vi "PlLoN_grabber.vi"(7 "Number of Images":u32=1 min=1 step=1, 8 "error in (no error)":errorcluster, 11 "Camera Handle":u32) -> (0 "error out":errorcluster, 1 "DATA":u16[][](array[numeric]), 2 "Number of Images":u32=1 min=1 step=1, 3 "Camera Handle":u32, 4 "x/y":dbl)   [LabVIEW 2015]
panel:
  out "Waveform Graph":u16[][](graph)
  out "PyLoN Ready":bool
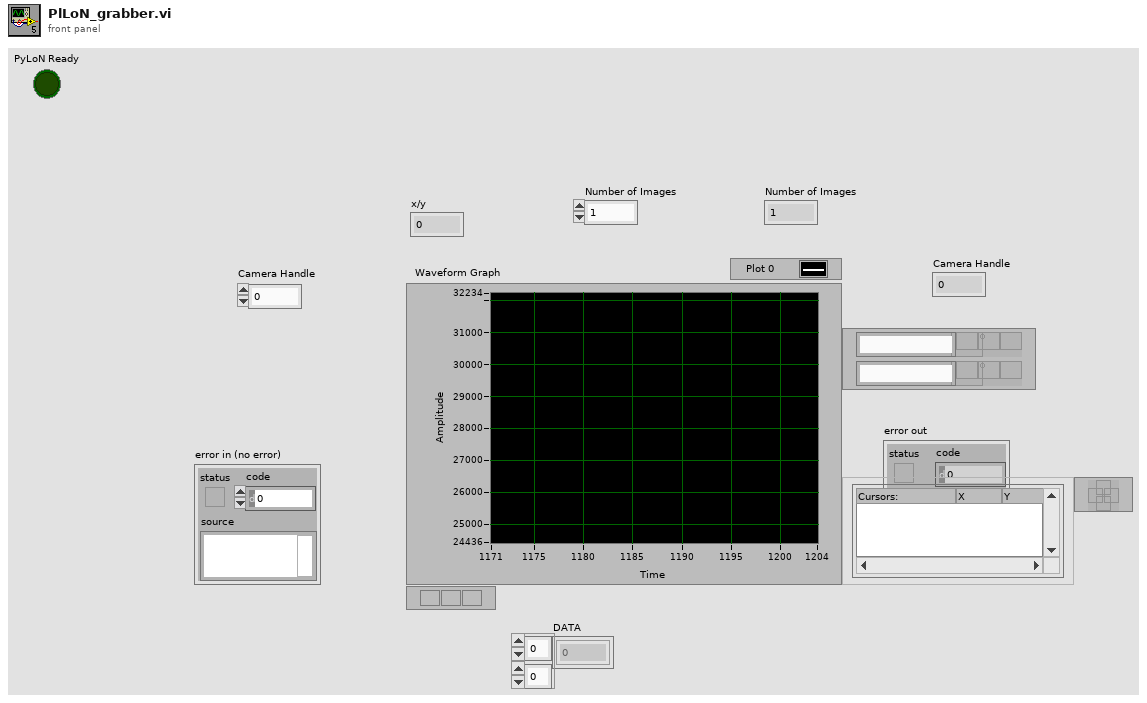
[diagram p1: front panel]
types:
  T1 = cluster{"acquire focus mode":u32, "Exposure Time (s)":dbl, "Number of Images":u32, "Software accumulation":u32}
  T2 = cluster{"Camera Handle":u32, "Pulser Handle":u32, "File Handle":u32, "Display Handle":u32, "Image Handle":u32}
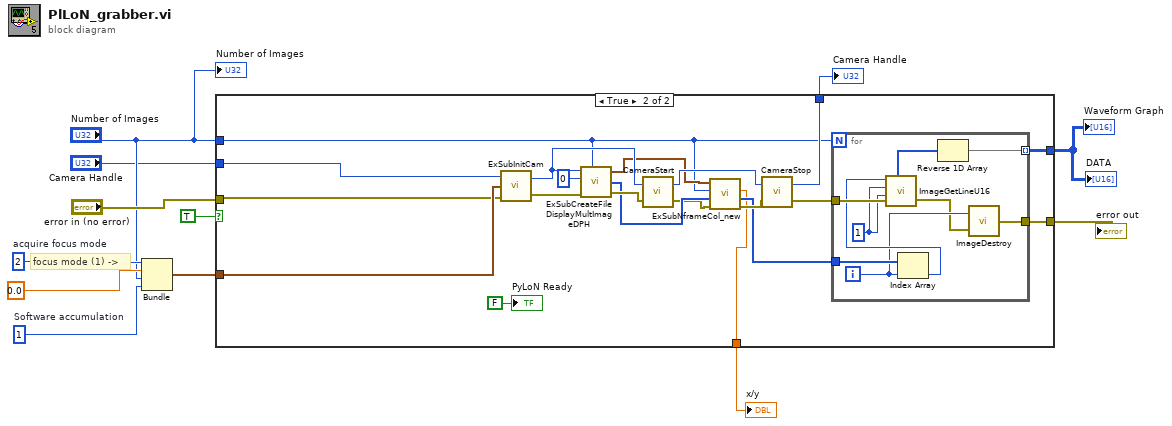
[diagram p0: block diagram]
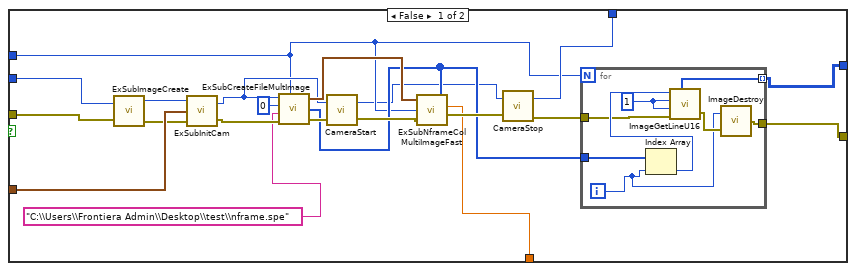
[diagram p2: hidden frame]
diagram:
  w6 = u32 2  # acquire focus mode
  w7 = u32 1  # Software accumulation
  # "focus mode (1) ->"
  n1 = Bundle("acquire focus mode"=w6, "Exposure Time (s)"=0.0, "Number of Images"="Number of Images", "Software accumulation"=w7) -> (w5:T1)  [unwired: 1 in]
  n2 = case shown="True" TRUE {
    tunnel: [w18 w58] -> w1
    tunnel: [w16 w57] -> w12
    tunnel: [w17 w52] -> w11
    tunnel: "Number of Images" -> [w14 w49]
    tunnel: [w15 w44] -> w10
    tunnel: "error in (no error)" -> [w33 w42]
    tunnel: w5 -> [w31 w51]
    tunnel: "Camera Handle" -> [w29 w43]
    frame False {
      n3 = call "ExSubImageCreate.vi"("Camera Handle"=w29, "error in (no error)"=w33) -> ("Camera Handle"=w32:u32, "error out"=w30:errorcluster)  [unwired: 1 out]
      n4 = call "ExSubInitCam.vi"("error in (no error)"=w30, "Camera Information"=w31, "Camera Handle"=w32) -> ("error out"=w28:errorcluster, "Camera Handle"=w22:u32)
      n5 = call "ExSubCreateFileMultImage.vi"("Camera Handle"=w22, "Pulser Handle"=u32 0, "File and Display Name"="C:\\Users\\Frontiera Admin\\Desktop\\test\\nframe.spe", "error in (no error)"=w28, "Number of Images"=w14) -> ("Handles Out"=w23:T2, "Array"=w20:u32[], "error out"=w25:errorcluster)
      n6 = call <userlib>:"CameraStart.vi"("error in"=w25, "Camera Handle"=w22) -> ("error out"=w24:errorcluster, "Camera Handle"=w13:u32)
      n7 = call "ExSubNframeColMultiImageFast.vi"("Handle Cluster"=w23, "Number of Images"=w14, "error in (no error)"=w24, "image handles"=w20) -> ("x/y"=w15:dbl, "error out"=w21:errorcluster)  [unwired: 1 out]
      n8 = call <userlib>:"CameraStop.vi"("error in"=w21, "Camera Handle"=w13) -> ("error out"=w19:errorcluster, "Camera Handle"=w16:u32)
      n9 = for {
        N: w14 -> [_]
        tunnel: w20 -> [w41]
        tunnel: w19 -> [w38]
        tunnel: [w37] -> w18 mode=indexing
        tunnel: [w35] -> w17
        i -> [w34]
        w39 = u32 1 ("Y Position")
        n10 = Index Array(array=w41, index=w34) -> (element=w40:u32)
        n11 = call <userlib>:"ImageGetLineU16.vi"("Data Handle"=w40, "Y Position"=w39, "Z Position"=w39, "error in"=w38) -> ("Array u16"=w37:u16[], "error out"=w36:errorcluster)  [unwired: 1 out]
        n12 = call <userlib>:"ImageDestroy.vi"("error in"=w36, "Data handle"=w34) -> ("error out"=w35:errorcluster)
      }
    }
    frame True {
      n13 = call "ExSubInitCam.vi"("error in (no error)"=w42, "Camera Information"=w51, "Camera Handle"=w43) -> ("error out"=w56:errorcluster, "Camera Handle"=w54:u32)
      n14 = call "ExSubCreateFileDisplayMultImageDPH.vi"("Camera Handle"=w54, "Pulser Handle"=u32 0, "error in (no error)"=w56, "Number of Images"=w49) -> ("Handles Out"=w50:T2, "Array"=w48:u32[], "error out"=w55:errorcluster)  [unwired: 1 in]
      n15 = call <userlib>:"CameraStart.vi"("error in"=w55, "Camera Handle"=w54) -> ("error out"=w47:errorcluster, "Camera Handle"=w59:u32)
      n16 = call "ExSubNframeCol_new.vi"("error in (no error)"=w47, "image handles"=w48, "Number of Images"=w49, "Handle Cluster 2"=w50) -> ("error out"=w46:errorcluster, "data handles"=w45:u32[], "x/y"=w44:dbl)  [unwired: 4 in, 1 out]
      n17 = call <userlib>:"CameraStop.vi"("error in"=w46, "Camera Handle"=w59) -> ("error out"=w60:errorcluster, "Camera Handle"=w57:u32)
      n18 = for {
        N: w49 -> [_]
        tunnel: w45 -> [w67]
        tunnel: w60 -> [w70]
        tunnel: [w62] -> w58 mode=indexing
        tunnel: [w64] -> w52
        i -> [w66]
        w69 = u32 1
        n19 = Index Array(array=w67, index=w66) -> (element=w68:u32)
        n20 = call <userlib>:"ImageGetLineU16.vi"("Data Handle"=w68, "Y Position"=w69, "Z Position"=w69, "error in"=w70) -> ("Array u16"=w63:u16[], "error out"=w65:errorcluster)  [unwired: 1 out]
        n21 = Reverse 1D Array(array=w63) -> (reversed array=w62:u16[])
        n22 = call <userlib>:"ImageDestroy.vi"("error in"=w65, "Data handle"=w66) -> ("error out"=w64:errorcluster)
      }
      "PyLoN Ready" <- FALSE ("PyLoN Ready")
    }
  }
  "error out" <- w11
  "DATA" <- w1
  "Camera Handle" <- w12
  "x/y" <- w10
  "Waveform Graph" <- w1
  "Number of Images" <- "Number of Images"
